vi "Load Class From File on Disk.vi"(8 "error in (no error)":errorcluster, 10 "File Path Control":path, 11 "Abstract Spectrometer in":refnum<class "Abstract Spectrometer.lvclass">) -> (0 "error out":errorcluster, 3 "specific class reference":refnum<class "Abstract Spectrometer.lvclass">)   [LabVIEW 2019]
uses:
  Abstract Spectrometer.lvclass
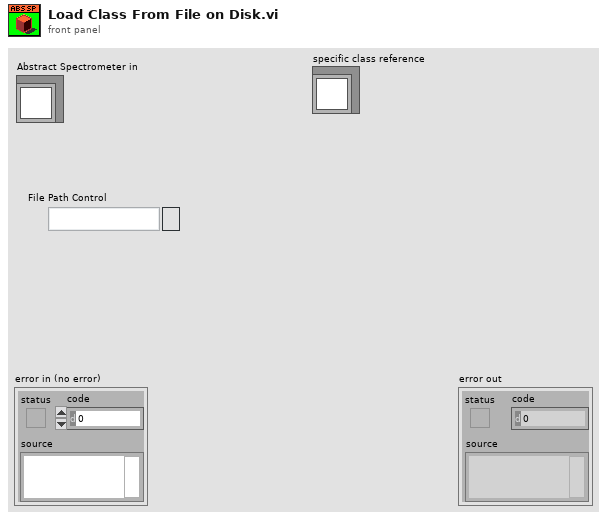
[diagram p1: front panel]
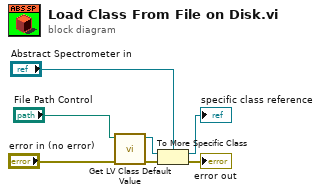
[diagram p0: block diagram]
diagram:
  n1 = call <vilib>:"Get LV Class Default Value.vi"("error in (no error)"="error in (no error)", "class path"="File Path Control") -> ("error out"=w4:errorcluster, "object"=w5:refnum<class>)  [unwired: 8 in]
  n2 = To More Specific Class(target class="Abstract Spectrometer in", reference=w5, error in=w4) -> (specific class reference=→"specific class reference":refnum<class "Abstract Spectrometer.lvclass">, error out=→"error out":errorcluster)
